vi "Write New Message Msg.vi"(10 "WebSocket Client.lvlib:New Message Msg.lvclass":refnum<class "New Message Msg.lvclass">, 11 "WebSocket Client in":refnum<class "WebSocket Client.lvclass">) -> (3 "WebSocket Client out":refnum<class "WebSocket Client.lvclass">)   [LabVIEW 2017, in "WebSocket Client.lvlib" / "WebSocket Client.lvclass"]
uses:
  WebSocket Client.lvclass
  WebSocket Client Messages/New Message Msg/New Message Msg.lvclass
  WebSocket Client.lvclass/WebSocket Client.ctl
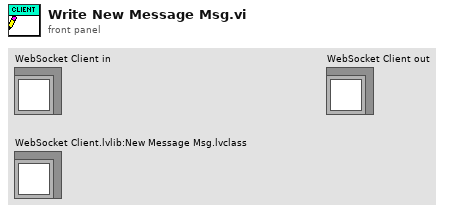
[diagram p1: front panel]
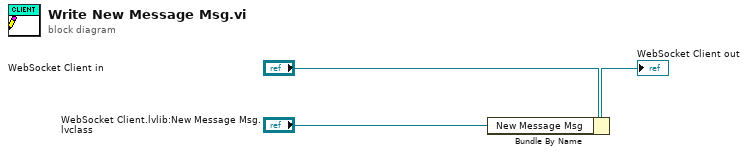
[diagram p0: block diagram]
diagram:
  n1 = Bundle By Name(cluster="WebSocket Client in", "New Message Msg"="WebSocket Client.lvlib:New Message Msg.lvclass") -> (→"WebSocket Client out":refnum<class "WebSocket Client.lvclass">)
